vi "Banda Transportadora.vi"() -> ()   [LabVIEW 2019]
panel:
  in  "Banda Transportadora":dbl(slide) scale=0.0..1200.0
  in  "Dirección":bool=TRUE
  in  "Velocidad (m/300ms)":dbl(knob)=1.0 scale=0.0..10.0 scale format="%#_2g"
  out "Tope Izquierdo":bool
  out "Tope Derecho":bool
  in  "stop":bool
  in  "Acción":bool=TRUE
  # "Continuar"
  # "Derecha"
  # "Detener"
  # "Izquierda"
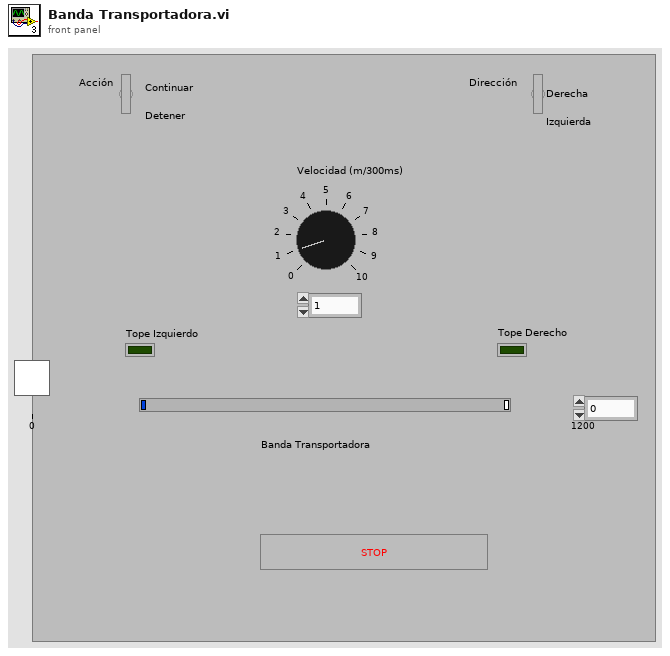
[diagram p1: front panel]
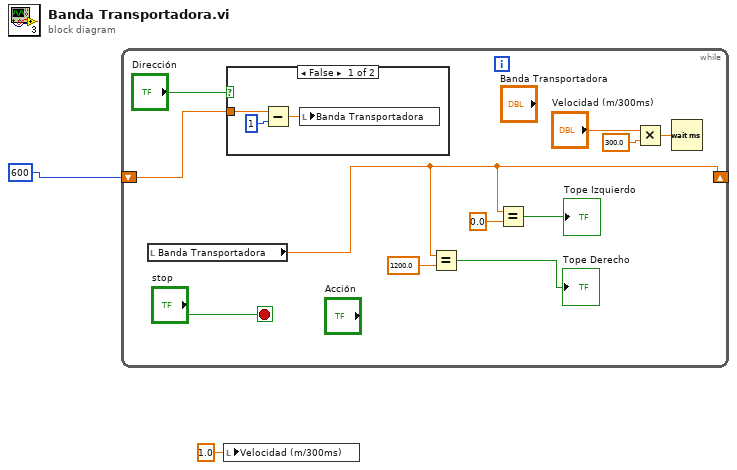
[diagram p0: block diagram]
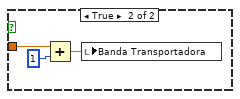
[diagram p2: hidden frame]
diagram:
  n1 = while {
    shift-right: [w4] -> _
    shift-left: 600 -> [w8]
    stop <- "stop" stop-if-true
    n2 = local read "Banda Transportadora"() -> (w4:dbl)
    n3 = case shown="False" "Dirección" {
      tunnel: w8 -> [w16 w19]
      frame False {
        n4 = Subtract(x=w16, y=1) -> (x-y=w14:dbl)
        n5 = local write "Banda Transportadora"(w14) -> ()
      }
      frame True {
        n6 = Add(x=w19, y=1) -> (x+y=w17:dbl)
        n7 = local write "Banda Transportadora"(w17) -> ()
      }
    }
    n8 = Equal?(x=w4, y=1200.0) -> (x = y?=→"Tope Derecho":bool)
    n9 = Equal?(x=w4, y=0.0) -> (x = y?=→"Tope Izquierdo":bool)
    n10 = Multiply(x="Velocidad (m/300ms)", y=300.0) -> (x*y=w10:dbl)
    n11 = Wait (ms)(milliseconds to wait=w10) -> ()  [unwired: 1 out]
  }
  n12 = local write "Velocidad (m/300ms)"(1.0 ("Velocidad (m/300ms)")) -> ()
